vi "Write Multiple Coils1.vi"(7 "Unit_ID":T1={"Protocol ID"=0, "Unit ID"=1}, 8 "error in (no error)":errorcluster, 9 "coil values":bool[](array[boolean]), 10 "starting address":u16, 11 "Modbus master in":refnum<class "TCP.lvclass">) -> (0 "error out":errorcluster, 3 "Modbus master out":refnum<class "TCP.lvclass">)   [LabVIEW 2019, in "NI_modbus_upd.lvlib"]
doc: "Writes values to contiguous coils. The maximum number of coils this VI can write is 1,968."
uses:
  NI_modbus_upd.lvlib
  TCP/TCP.lvclass
  Ctl/Unit_ID.ctl
  TCP/TCP.lvclass/TCP.ctl
  Error Generator1.vi
  Function code mismatch error1.vi
  Read ADU Packet Master.vi
  Write ADU Packet Master.vi
  Modbus Data Unit (PDU)/Construct PDU1.vi
  Utility/Bits to Bytes1.vi
  Modbus Data Unit (PDU)/Unflatten to PDU1.vi
  TCP/Protocol Read.vi
  TCP/Protocol Write.vi
  <vilib>/Utility/error.llb/Clear Errors.vi
  Modbus Data Unit (PDU)/Deconstruct PDU1.vi
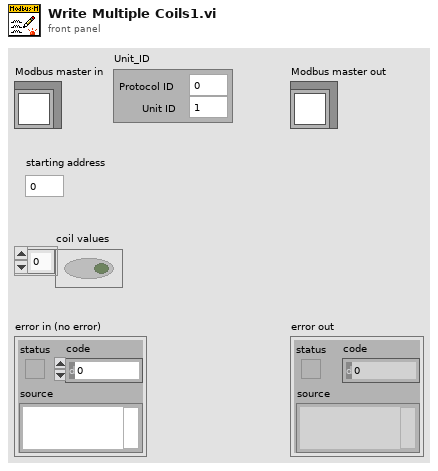
[diagram p1: front panel]
types:
  T1 = typedef "NI_modbus_upd.lvlib/Unit_ID.ctl" = cluster{"Protocol ID":u16, "Unit ID":u8}
  T2 = typedef "NI_modbus_upd.lvlib/MB Modbus Data Unit.ctl" = cluster{"function":T3, "Data":u8[]}
  T3 = typedef "NI_modbus_upd.lvlib/Function.ctl" = u8
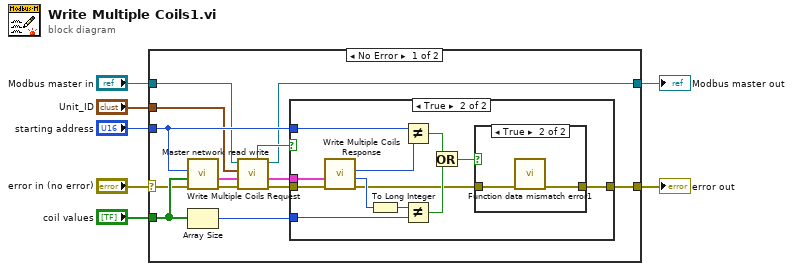
[diagram p0: block diagram]
diagram:
  n1 = case shown="No Error" "error in (no error)" {
    selector: "error in (no error)" -> [w8 w38]
    tunnel: "Modbus master in" -> [w11 w37]
    tunnel: [w19 w38] -> w6
    tunnel: [w13 w37] -> w7
    tunnel: "starting address" -> [w18 _]
    tunnel: "coil values" -> [w17 _]
    tunnel: "Unit_ID" -> [w10 _]
    frame No Error {
      n2 = call "Write Multiple Coils Request.vi"("error in (no error)"=w8, "coils to write"=w17, "starting address"=w18) -> ("error out"=w20:errorcluster, "Modbus Data Unit out"=w12:T2)  [unwired: 7 in]
      n3 = Array Size(array=w17) -> (size(s)=w16:i32)
      n4 = call "Master network read write.vi"("error in (no error)"=w20, "Modbus Data Unit"=w12, "Unit_ID"=w10, "TCP in"=w11) -> ("error out"=w15:errorcluster, "Modbus data unit out"=w9:T2, "TCP out"=w13:refnum<class "TCP.lvclass">, "PDU valid?"=w14:bool)  [unwired: 4 in]
      n5 = case shown="True" w14 {
        tunnel: [w21 w30] -> w19
        tunnel: w18 -> [_ w24]
        tunnel: w16 -> [_ w28]
        tunnel: w15 -> [w21 w27]
        tunnel: w9 -> [_ w22]
        frame False {
        }
        frame True {
          n6 = call "Write Multiple Coils Response.vi"("error in (no error)"=w27, "Modbus Data Unit in"=w22) -> ("error out"=w26:errorcluster, "number of coils"=w29:u16, "start address"=w25:u16)  [unwired: 7 in]
          n7 = To Long Integer(number=w29) -> (32bit integer=w23:i32)
          n8 = Not Equal?(x=w24, y=w25) -> (x != y?=w32:bool)
          n9 = Not Equal?(x=w23, y=w28) -> (x != y?=w31:bool)
          n10 = Or(x=w32, y=w31) -> (x .or. y?=w33:bool)
          n11 = case shown="True" w33 {
            tunnel: [w34 w35] -> w30
            tunnel: w26 -> [w34 w36]
            frame False {
            }
            frame True {
              n12 = call "Function data mismatch error1.vi"("error in (no error)"=w36) -> ("error out"=w35:errorcluster)  [unwired: 10 in]
            }
          }
        }
      }
    }
    frame Error {
    }
  }
  "error out" <- w6
  "Modbus master out" <- w7
